vi "build_set_preregistration_data_msg.vi"(8 "error_in":errorcluster, 11 "preregistration_data":T1 {"Starting serial number" format="%#_11g"}) -> (0 "error_out":errorcluster, 3 "command":string)   [LabVIEW 2018]
uses:
  controls/preregistration_data.ctl
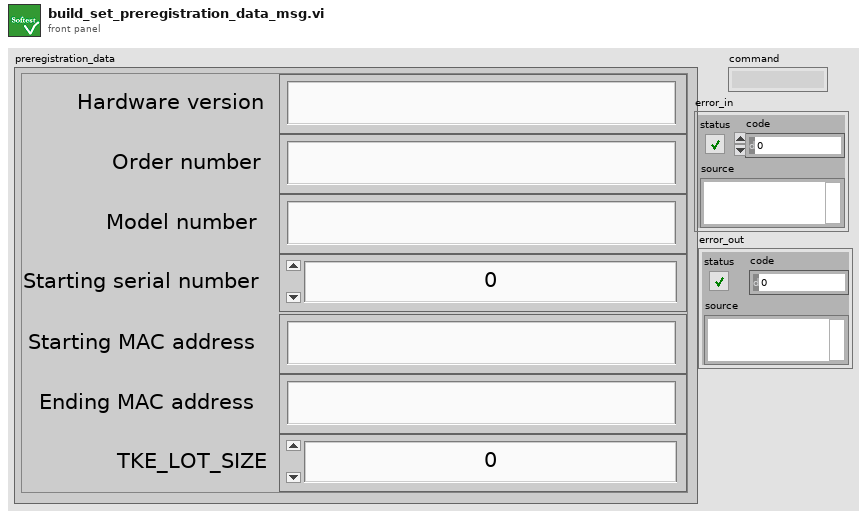
[diagram p1: front panel]
types:
  T1 = typedef "preregistration_data.ctl" = cluster{"Hardware version":string, "Order number":string, "Model number":string, "Starting serial number":i32, "Starting MAC address":string, "Ending MAC address":string, "TKE_LOT_SIZE":i32}
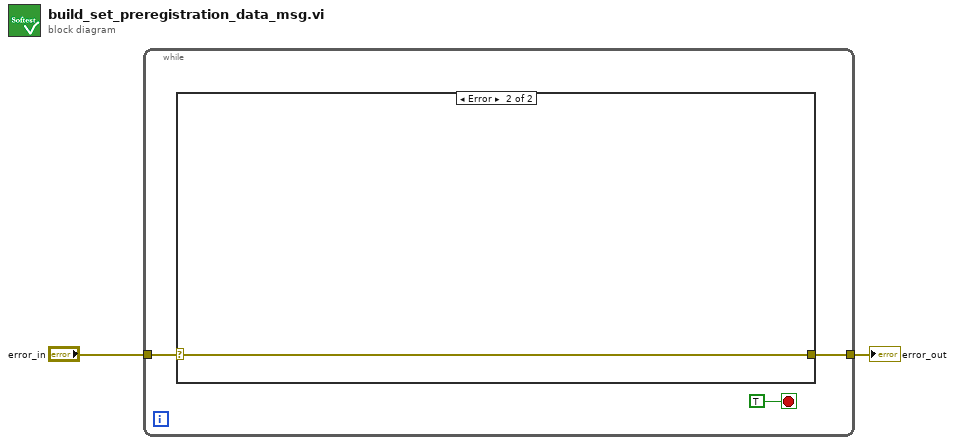
[diagram p0: block diagram]
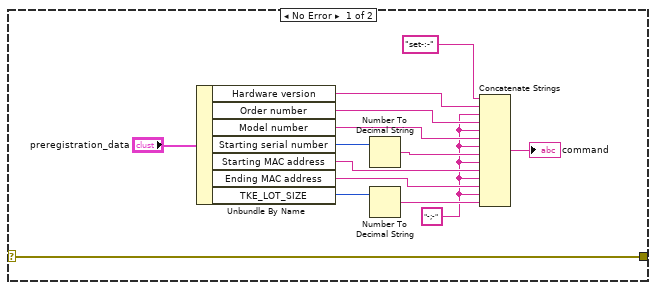
[diagram p2: hidden frame]
diagram:
  n1 = while {
    tunnel: "error_in" -> [w4]
    tunnel: [w3] -> w1
    stop <- TRUE stop-if-true
    n2 = case shown="Error" w4 {
      selector: w4 -> [w6 w20]
      tunnel: [w6 w20] -> w3
      frame No Error {
        w7 = "-;-" ("string")
        n3 = Unbundle By Name("preregistration_data") -> ("Hardware version"=w17:string, "Order number"=w13:string, "Model number"=w12:string, "Starting serial number"=w15:i32, "Starting MAC address"=w10:string, "Ending MAC address"=w9:string, "TKE_LOT_SIZE"=w14:i32)
        n4 = Number To Decimal String(number=w15) -> (decimal integer string=w11:string)  [unwired: 1 in]
        n5 = Number To Decimal String(number=w14) -> (decimal integer string=w8:string)  [unwired: 1 in]
        n6 = Concatenate Strings("set-:-" ("string"), w17, w7, w13, w7, w12, w7, w11, w7, w10, w7, w9, w7, w8) -> (→"command":string)
      }
      frame Error {
      }
    }
  }
  "error_out" <- w1
